vi "CreateNotifier.vi"(8 "error in (no error)":errorcluster, 11 "ByRefClass in":refnum<class "ClassByRef.lvclass">) -> (0 "error out":errorcluster, 2 "notifier out":refnum<notifier>, 3 "ByRefClass out":refnum<class "ClassByRef.lvclass">)   [LabVIEW 2021, in "ClassUtilities.lvlib" / "ClassByRef.lvclass"]
uses:
  ClassByRef.lvclass
  ClassByRef.lvclass/ClassByRef.ctl
  SetNotifier.vi
  SetNotifier.vi/6a7be9d6-cac5-4ac9-b7fd-da113b1d2d73.vi
  GetRef.vi
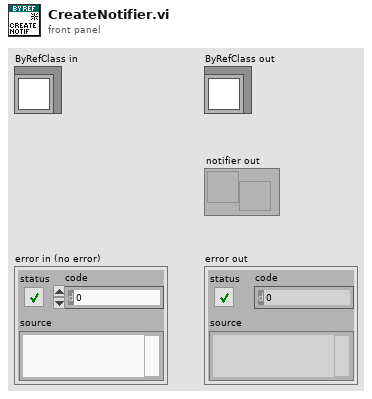
[diagram p1: front panel]
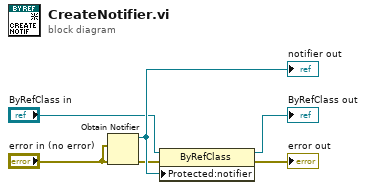
[diagram p0: block diagram]
diagram:
  n1 = Obtain Notifier(notification data type="error in (no error)", error in (no error)="error in (no error)") -> (notifier out=w6:refnum<notifier>, error out=w2:errorcluster)  [unwired: 2 in, 1 out]
  "notifier out" <- w6
  n2 = property class="ByRefClass"(reference="ByRefClass in", error in=w2, "Protected:notifier"=w6) -> (reference out=→"ByRefClass out":refnum<class "ClassByRef.lvclass">, error out=→"error out":errorcluster)
